vi "openZCANPRO.vi"   [LabVIEW 2015]
uses:
  <vilib>/registry/registry.llb/Registry RtKey.ctl
  <vilib>/registry/registry.llb/Registry SAM.ctl
  <vilib>/registry/registry.llb/Registry View.ctl
  <vilib>/registry/registry.llb/Read Registry Value Simple STR.vi
  <vilib>/Platform/browser.llb/Open URL in Default Browser (string).vi
types:
  T1 = typedef "Registry View.ctl" = u16
  T2 = typedef "Registry SAM.ctl" = enum32{"KEY_QUERY_VALUE", "KEY_SET_VALUE", "KEY_CREATE_SUB_KEY", "KEY_ENUMERATE_SUB_KEYS", "KEY_NOTIFY", "KEY_CREATE_LINK", "KEY_READ", "KEY_WRITE", "KEY_ALL_ACCESS", "KEY_READ | KEY_WRITE"}
  T3 = typedef "Registry RtKey.ctl" = enum32{"HKEY_CLASSES_ROOT", "HKEY_CURRENT_USER", "HKEY_LOCAL_MACHINE", "HKEY_USERS", "HKEY_PERFORMANCE_DATA", "HKEY_CURRENT_CONFIG", "HKEY_DYN_DATA"}
  T4 = typedef "Registry refnum.ctl" = refnum<k1>
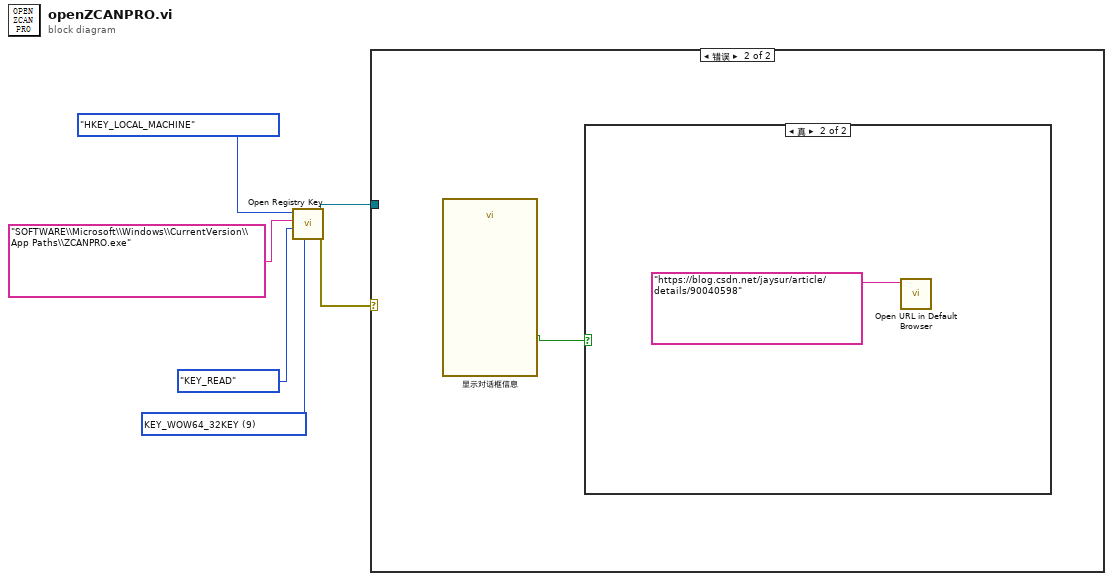
[diagram p0: block diagram]
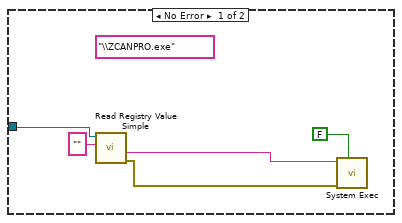
[diagram p2: hidden frame]
diagram:
  w3 = T1 9 items=["Default"=0, "KEY_WOW64_64KEY"=8, "KEY_WOW64_32KEY"=9] ("registry view")
  n1 = call <vilib>:"Open Registry Key.vi"("registry view"=w3, "security access mask (KEY_READ | KEY_WRITE)"=Registry_SAM."KEY_READ", "subkey"="SOFTWARE\\Microsoft\\Windows\\CurrentVersion\\App Paths\\ZCANPRO.exe", "root key (HKEY_LOCAL_MACHINE)"=Registry_RtKey."HKEY_LOCAL_MACHINE") -> ("error out"=w1:errorcluster, "refnum out"=w2:T4)  [unwired: 6 in]
  n2 = case shown="错误" w1 {
    tunnel: w2 -> [w9 _]
    frame No Error {
      (unwired) "\\ZCANPRO.exe" ("字符串")
      n3 = call-poly <vilib>:"Read Registry Value Simple.vi"("value"="", "refnum"=w9) -> ("error out"=w10:errorcluster, "String/Binary data"=w8:string)  [unwired: 4 in, 2 out]
      n4 = call <vilib>:"System Exec.vi"("wait until completion? (T)"=FALSE, "error in (no error)"=w10, "command line"=w8) -> ()  [unwired: 5 in, 4 out]
    }
    frame Error {
      n5 = call "显示对话框信息"() -> ("前往下载"=w12:bool)  [unwired: 10 in, 1 out]
      n6 = case shown="真" w12 {
        frame False {
        }
        frame True {
          n7 = call-poly <vilib>:"Open URL in Default Browser.vi"("URL"="https://blog.csdn.net/jaysur/article/details/90040598") -> ()  [unwired: 5 in, 2 out]
        }
      }
    }
  }
